vi "test3-ProcessAsyncMessageWithoutReplyInCSMLoop(SendAndReceive).vi"(8 "error in (no error)":errorcluster, 11 "TestCase in":refnum<class "testcase-CSMAddonLoopSupport.lvclass">) -> (0 "error out":errorcluster, 3 "TestCase out":refnum<class "testcase-CSMAddonLoopSupport.lvclass">)   [LabVIEW 2017, in "testcase-CSMAddonLoopSupport.lvclass"]
uses:
  testcase-CSMAddonLoopSupport.lvclass
  4585ddd5-ba69-4fd4-94fe-207595864cbd.vi
  a7620e19-6451-46a1-85ca-ade5edb58587.vi
  55fec5d7-cd22-46f7-b641-2c7c49619fc8.vi
  9cfd6824-310a-46c9-9b98-3854de5c7aa2.vi
  <vilib>/addons/_JKI Toolkits/VI Tester/TestCase.llb/TestCase.lvclass
  src/user.lib/_NEVSTOP/Communicable State Machine(CSM)/Communicable State Machine.lvlib
  CSM/CSM-Testcase.lvlib
  C:/Program Files (x86)/National Instruments/LabVIEW 2017/vi.lib/addons/_JKI Toolkits/VI Tester/TestCase.llb/TestCase.lvclass
panel:
  out "LoopCount":i32
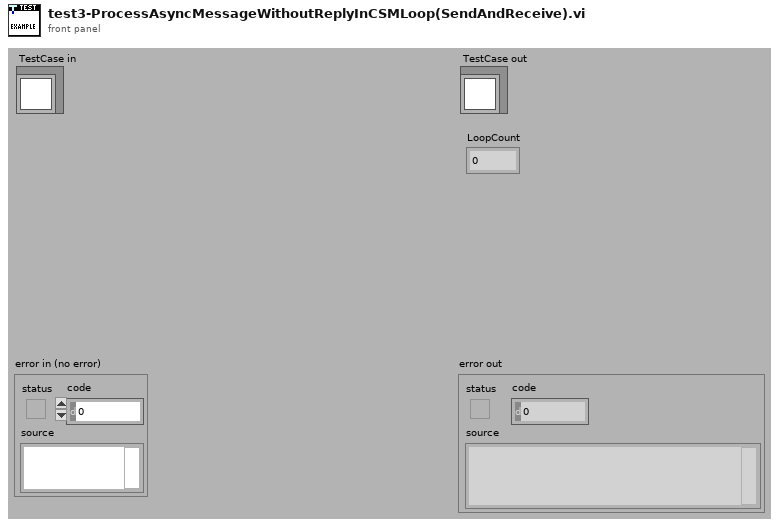
[diagram p1: front panel]
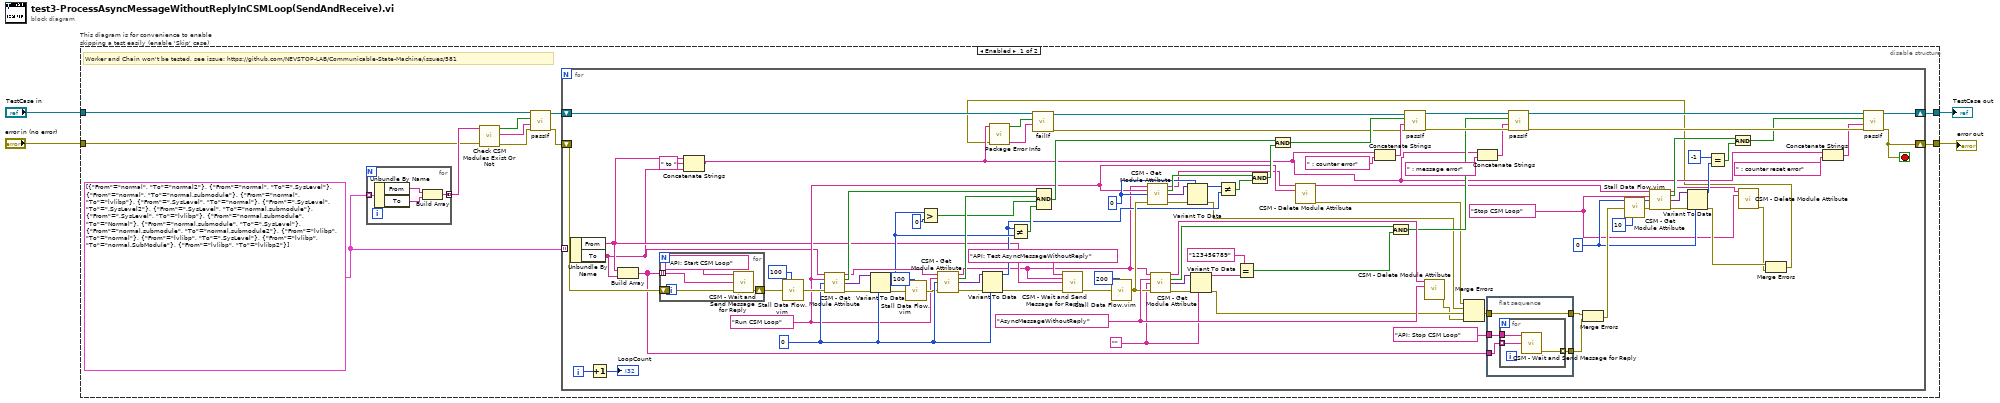
[diagram p0: block diagram]
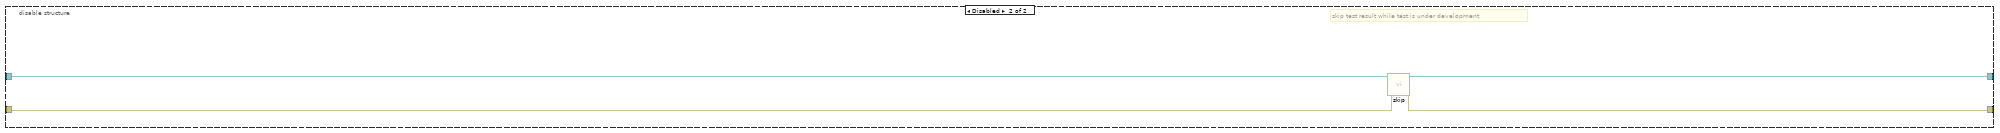
[diagram p2: hidden frame]
diagram:
  n1 = disable-structure "This diagram is for convenience to enable skipping a test easily (enable 'Skip' case)" shown="Enabled" {
    disable-tunnel: "TestCase in" -> [w6 w131]
    disable-tunnel: [w15 w129] -> w1
    disable-tunnel: [w14 w130] -> w3
    disable-tunnel: "error in (no error)" -> [w8 w128]
    frame Enabled {
      w9 = cluster{"From":string, "To":string}[] [{"From"="normal", "To"="normal2"}, {"From"="normal", "To"=".SysLevel"}, {"From"="normal", "To"="normal.submodule"}, {"From"="normal", "To"="lvlibp"}, {"From"=".SysLevel", "To"="normal"}, {"From"=".SysLevel", "To"=".SysLevel2"}, {"From"=".SysLevel", "To"="normal.submodule"}, {"From"=".SysLevel", "To"="lvlibp"}, {"From"="normal.submodule", "To"="Normal"}, {"From"="normal.submodule", "To"=".SysLevel"}, {"From"="normal.submodule", "To"="normal.submodule2"}, {"From"="lvlibp", "To"="normal"}, {"From"="lvlibp", "To"=".SysLevel"}, {"From"="lvlibp", "To"="normal.SubModule"}, {"From"="lvlibp", "To"="lvlibp2"}]
      # "Worker and Chain won't be tested, see issue: https://github.com/NEVSTOP-LAB/Communicable-State-Machine/issues/581"
      n2 = for {
        tunnel: w9 -> [w19] mode=indexing
        tunnel: [w16] -> w12 mode=concatenating
        n3 = Unbundle By Name(w19) -> ("From"=w18:string, "To"=w17:string)
        n4 = Build Array(w18, w17) -> (w16:string[])
      }
      n5 = call "Check CSM Modules Exist Or Not.vi"("error in"=w8, "CSM names in"=w12) -> ("error out"=w10:errorcluster, "Debug string"=w11:string, "All Modules Exist?"=w13:bool)  [unwired: 7 in]
      n6 = call-dynamic "passIf.vi"("error in (no error)"=w10, "message (\"\")"=w11, "pass"=w13, "TestCase in"=w6) -> ("error out"=w7:errorcluster, "TestCase out"=w5:refnum<class "testcase-CSMAddonLoopSupport.lvclass">)  [unwired: 6 in]
      n7 = for {
        tunnel: w9 -> [w44] mode=indexing
        shift-right: [w28] -> w15
        shift-left: w5 -> [w24]
        shift-right: [w27] -> w14
        shift-left: w7 -> [w70]
        i -> [w116]
        stop <- w27 stop-if-true
        w33 = ""
        w47 = "Stop CSM Loop" ("State")
        w60 = 0
        w80 = 0
        w94 = 0
        w51 = "Run CSM Loop" ("State")
        w105 = "AsyncMessageWithoutReply" ("State")
        n8 = Unbundle By Name(w44) -> ("From"=w42:string, "To"=w41:string)
        n9 = Increment(x=w116) -> (x+1=→"LoopCount":i32)
        n10 = Build Array(w42, w41) -> (w43:string[])
        n11 = for {
          shift-right: [w119] -> w114
          shift-left: w70 -> [w118]
          tunnel: w43 -> [w117] mode=indexing
          n12 = call "CSM - Wait and Send Message for Reply.vi"("State"="API: Start CSM Loop", "Target Module"=w117, "Error In (No Error)"=w118) -> ("error out"=w119:errorcluster)  [unwired: 9 in, 3 out]
        }
        n13 = Concatenate Strings(w42, " to " ("string"), w41) -> (w21:string)
        n14 = call "Stall Data Flow.vim"("value in"=w114, "milliseconds to wait"=u32 100) -> ("value out"=w102:errorcluster)  [unwired: 1 out]
        n15 = call "CSM - Get Module Attribute.vi"("CSM Name"=w41, "Attribute"=w51, "Default Value (Empty Variant)"=w94, "Error In"=w102) -> ("CSM Name (Dup)"=w96:string, "Found"=w101:bool, "Value"=w95:variant, "error out"=w99:errorcluster)  [unwired: 7 in, 1 out]
        n16 = Variant To Data(error in=w99, type=w94, Variant=w95) -> (data=w89:i32, error out=w88:errorcluster)
        n17 = call "Stall Data Flow.vim"("value in"=w88, "milliseconds to wait"=u32 100) -> ("value out"=w87:errorcluster)  [unwired: 1 out]
        n18 = Greater?(x=w89, y=0) -> (0:w92:bool)
        n19 = call "CSM - Get Module Attribute.vi"("CSM Name"=w96, "Attribute"=w51, "Default Value (Empty Variant)"=w94, "Error In"=w87) -> ("CSM Name (Dup)"=w29:string, "Found"=w100:bool, "Value"=w91:variant, "error out"=w98:errorcluster)  [unwired: 7 in, 1 out]
        n20 = Variant To Data(error in=w98, type=w94, Variant=w91) -> (data=w78:i32, error out=w97:errorcluster)
        n21 = Not Equal?(x=w78, y=w89) -> (x != y?=w90:bool)
        n22 = Compound Arithmetic op=AND(w101, w100, w92, w90) -> (w77:bool)
        n23 = call "CSM - Wait and Send Message for Reply.vi"("State"="API: Test AsyncMessageWithoutReply", "Arguments (\"\")"=w29, "Target Module"=w42, "Error In (No Error)"=w97) -> ("error out"=w110:errorcluster)  [unwired: 8 in, 3 out]
        n24 = call "Stall Data Flow.vim"("value in"=w110, "milliseconds to wait"=u32 200) -> ("value out"=w85:errorcluster)  [unwired: 1 out]
        n25 = call "CSM - Get Module Attribute.vi"("CSM Name"=w29, "Attribute"=w51, "Default Value (Empty Variant)"=w80, "Error In"=w85) -> ("CSM Name (Dup)"=w50:string, "Found"=w82:bool, "Value"=w81:variant, "error out"=w83:errorcluster)  [unwired: 7 in, 1 out]
        n26 = call "CSM - Get Module Attribute.vi"("CSM Name"=w29, "Attribute"=w105, "Default Value (Empty Variant)"=w33, "Error In"=w85) -> ("CSM Name (Dup)"=w106:string, "Found"=w107:bool, "Value"=w108:variant, "error out"=w109:errorcluster)  [unwired: 7 in, 1 out]
        n27 = Variant To Data(error in=w83, type=w80, Variant=w81) -> (data=w79:i32, error out=w49:errorcluster)
        n28 = Variant To Data(error in=w109, type=w33, Variant=w108) -> (data=w32:string, error out=w104:errorcluster)
        n29 = Not Equal?(x=w79, y=w78) -> (x != y?=w84:bool)
        n30 = Equal?(x="123456789", y=w32) -> (x = y?=w30:bool)
        n31 = Compound Arithmetic op=AND(w82, w84) -> (w76:bool)
        n32 = And(x=w77, y=w76) -> (x .and. y?=w75:bool)
        n33 = call "CSM - Delete Module Attribute.vi"("CSM Name"=w50, "Attribute"=w51) -> ("CSM Name (Dup)"=w46:string, "error out"=w48:errorcluster)  [unwired: 10 in, 2 out]
        n34 = Concatenate Strings(w21, " : counter error" ("format string")) -> (w38:string)
        n35 = And(x=w107, y=w30) -> (x .and. y?=w72:bool)
        n36 = call "CSM - Delete Module Attribute.vi"("CSM Name"=w106, "Attribute"=w105) -> ("error out"=w103:errorcluster)  [unwired: 10 in, 3 out]
        n37 = Merge Errors(w48, w49, w104, w103) -> (w52:errorcluster)
        n38 = Concatenate Strings(w21, " : message error" ("format string")) -> (w36:string)
        n39 = flat-sequence {
          tunnel: "API: Stop CSM Loop" ("State") -> [w124]
          tunnel: [w123] -> w67
          tunnel: [w122] -> w53
          tunnel: w52 -> [w122]
          tunnel: w43 -> [w121]
          frame #0 {
            n40 = for {
              tunnel: w124 -> [w127]
              tunnel: [w126] -> w123 mode=indexing
              tunnel: w121 -> [w125] mode=indexing
              n41 = call "CSM - Wait and Send Message for Reply.vi"("State"=w127, "Target Module"=w125) -> ("error out"=w126:errorcluster)  [unwired: 10 in, 3 out]
            }
          }
        }
        n42 = Merge Errors(w53, w67) -> (w65:errorcluster)
        n43 = call "Stall Data Flow.vim"("value in"=w65, "milliseconds to wait"=u32 10) -> ("value out"=w64:errorcluster)  [unwired: 1 out]
        n44 = call "CSM - Get Module Attribute.vi"("CSM Name"=w46, "Attribute"=w47, "Default Value (Empty Variant)"=w60, "Error In"=w64) -> ("CSM Name (Dup)"=w45:string, "Found"=w63:bool, "Value"=w61:variant, "error out"=w62:errorcluster)  [unwired: 7 in, 1 out]
        n45 = Variant To Data(error in=w62, type=w60, Variant=w61) -> (data=w59:i32, error out=w55:errorcluster)
        n46 = Equal?(x=-1, y=w59) -> (x = y?=w56:bool)
        n47 = And(x=w63, y=w56) -> (x .and. y?=w57:bool)
        n48 = call "CSM - Delete Module Attribute.vi"("CSM Name"=w45, "Attribute"=w47) -> ("error out"=w54:errorcluster)  [unwired: 10 in, 3 out]
        n49 = Merge Errors(w55, w54) -> (w20:errorcluster)
        n50 = call "Package Error Info.vi"("error in"=w20, "String in"=w21) -> ("packed error info out"=w25:string, "error status"=w26:bool)  [unwired: 8 in]
        n51 = call-dynamic "failIf.vi"("message (\"\")"=w25, "fail"=w26, "TestCase in"=w24) -> ("error out"=w22:errorcluster, "TestCase out"=w23:refnum<class "testcase-CSMAddonLoopSupport.lvclass">)  [unwired: 7 in]
        n52 = call-dynamic "passIf.vi"("error in (no error)"=w22, "message (\"\")"=w38, "pass"=w75, "TestCase in"=w23) -> ("error out"=w73:errorcluster, "TestCase out"=w74:refnum<class "testcase-CSMAddonLoopSupport.lvclass">)  [unwired: 6 in]
        n53 = call-dynamic "passIf.vi"("error in (no error)"=w73, "message (\"\")"=w36, "pass"=w72, "TestCase in"=w74) -> ("error out"=w68:errorcluster, "TestCase out"=w69:refnum<class "testcase-CSMAddonLoopSupport.lvclass">)  [unwired: 6 in]
        n54 = Concatenate Strings(w21, " : counter reset error" ("format string")) -> (w34:string)
        n55 = call-dynamic "passIf.vi"("error in (no error)"=w68, "message (\"\")"=w34, "pass"=w57, "TestCase in"=w69) -> ("error out"=w27:errorcluster, "TestCase out"=w28:refnum<class "testcase-CSMAddonLoopSupport.lvclass">)  [unwired: 6 in]
      }
    }
    frame Disabled {
      # "skip test result while test is under development"
      n56 = call <vilib>:"skip.vi"("error in (no error)"=w128, "TestCase in"=w131) -> ("error out"=w130:errorcluster, "TestCase out"=w129:refnum<class "testcase-CSMAddonLoopSupport.lvclass">)  [unwired: 8 in]
    }
  }
  "error out" <- w3
  "TestCase out" <- w1
